vi "StringJoiner.vi"(1 "string 2":string, 2 "string 1":string) -> (0 "concatenated string":string)   [LabVIEW 2010]
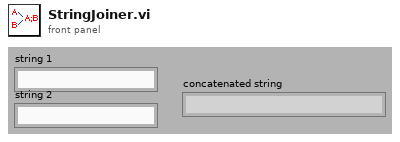
[diagram p1: front panel]
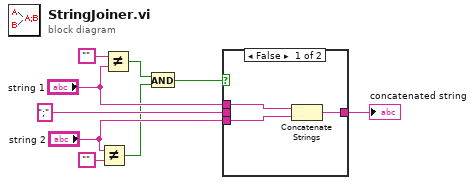
[diagram p0: block diagram]
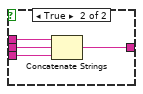
[diagram p2: hidden frame]
diagram:
  n1 = Not Equal?(x="string 2", y="") -> (x != y?=w1:bool)
  n2 = Not Equal?(x="", y="string 1") -> (x != y?=w7:bool)
  n3 = And(x=w7, y=w1) -> (x .and. y?=w4:bool)
  n4 = case shown="False" w4 {
    tunnel: ";" ("string") -> [_ w16]
    tunnel: [w10 w15] -> w8
    tunnel: "string 1" -> [w11 w14]
    tunnel: "string 2" -> [w12 w13]
    frame False {
      n5 = Concatenate Strings(w11, w12) -> (w10:string)
    }
    frame True {
      n6 = Concatenate Strings(w14, w16, w13) -> (w15:string)
    }
  }
  "concatenated string" <- w8
